vi "GuiRepository.vi"(0 "reference in":refnum<class "RemoteControl.lvclass">, 1 "Action(ReadRepository)":T1(ring), 5 "error in (no error)":errorcluster) -> (7 "QueueFromProcess":refnum<queue>, 9 "ProcessViRef":refnum<vi>, 11 "ProcessSyncQueue":refnum<queue>, 13 "EventFromProcess":refnum<user-event>, 14 "reference out":refnum<class "RemoteControl.lvclass">, 15 "EventsToProcess":refnum<user-event>, 17 "ProcessAlreadyStarted":bool, 19 "error out":errorcluster)   [LabVIEW 2012, in "RemoteControl.lvclass"]
uses:
  RemoteControl.lvclass
  Gui.ctl
  RemoteControl.lvclass/RemoteControl.ctl
  Gui.vi
panel:
  # "Use this indicator for sending messages to the Process VI"
  # "These indicators are used by the process VIs"
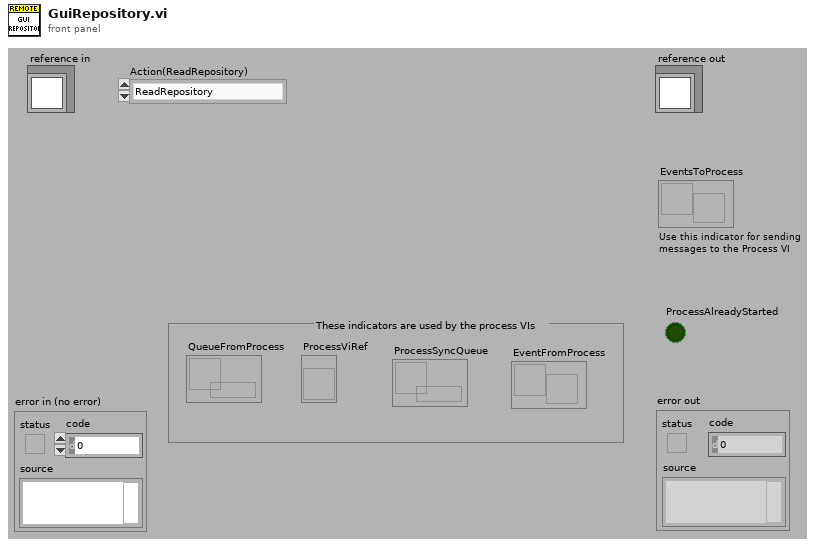
[diagram p1: front panel]
types:
  T1 = enum16{"ReadRepository", "CreateNew", "CreateOrLookUpExisting"}
  T2 = typedef "RemoteControl.lvclass/Gui.ctl" = cluster{"EventsToProcess":refnum<user-event>, "EventFromProcess":refnum<user-event>, "ProcessSyncQueue":refnum<queue>, "ProcessViRef":refnum<vi>, "QueueFromProcess":refnum<queue>}
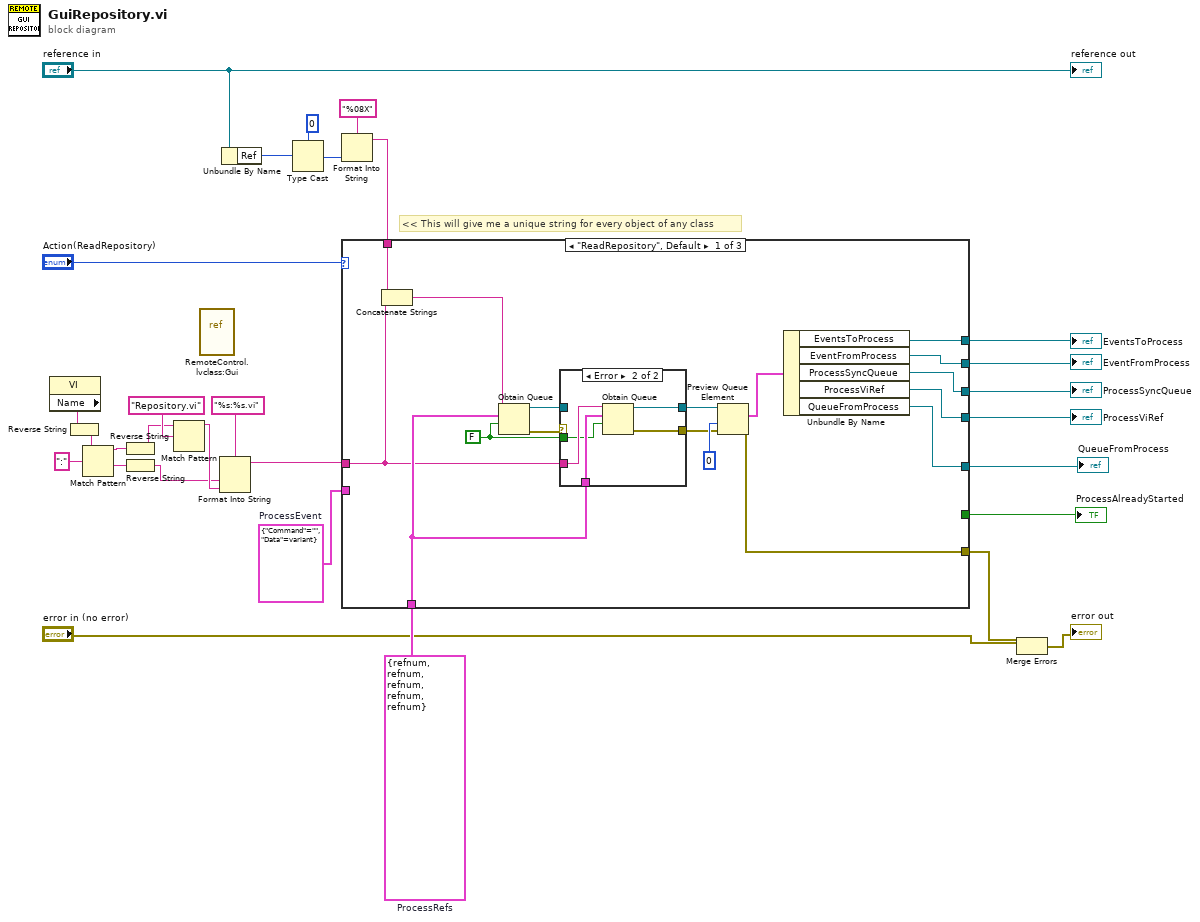
[diagram p0: block diagram]
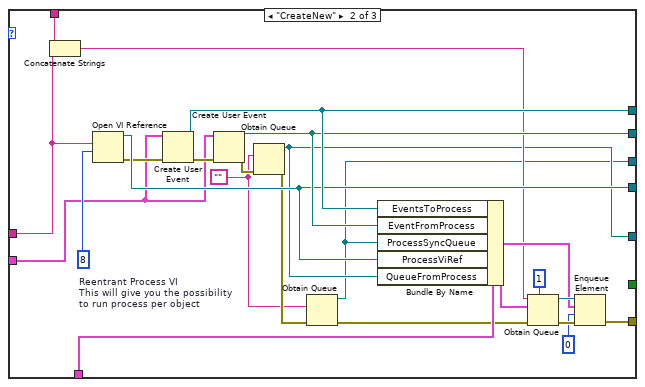
[diagram p3: hidden frame]
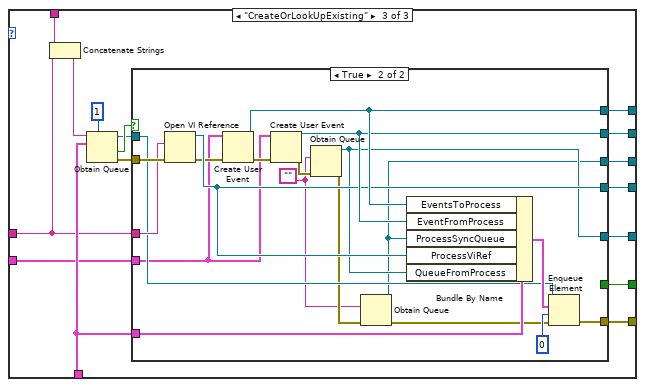
[diagram p4: hidden frame]
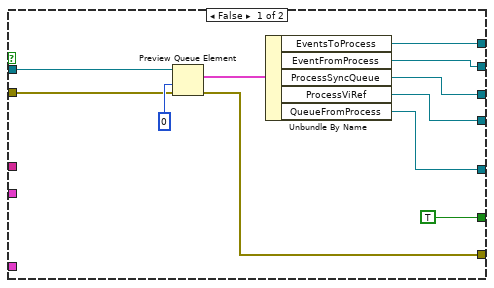
[diagram p5: hidden frame]
diagram:
  w13 = T2 {"EventsToProcess"=refnum, "EventFromProcess"=refnum, "ProcessSyncQueue"=refnum, "ProcessViRef"=refnum, "QueueFromProcess"=refnum}  # ProcessRefs
  w14 = cluster{"Command":string, "Data":variant} {"Command"="", "Data"=variant}  # ProcessEvent
  # "<< This will give me a unique string for every object of any class"
  n1 = property class="VI"() -> ("Name"=w20:string)  [unwired: 2 in, 2 out]
  n2 = Reverse String(1:w20) -> (0:w21:string)
  n3 = Match Pattern(string=w21, regular expression=":") -> (before substring=w25:string, after substring=w22:string)  [unwired: 1 in, 2 out]
  n4 = Reverse String(1:w25) -> (0:w26:string)
  n5 = Reverse String(1:w22) -> (0:w24:string)
  n6 = Match Pattern(string=w26, regular expression="Repository.vi") -> (before substring=w28:string)  [unwired: 1 in, 3 out]
  n7 = vi-ref "RemoteControl.lvclass:Gui.vi"() -> ()  [unwired: 1 out]
  n8 = Format Into String(format string="%s:%s.vi", w24, w28) -> (resulting string=w3:string)  [unwired: 2 in, 1 out]
  n9 = Unbundle By Name("reference in") -> ("Ref"=w15:u32)
  n10 = Type Cast(type=u32 0, x=w15) -> (*(type *) &x=w18:u32)
  n11 = Format Into String(format string="%08X", w18) -> (resulting string=w5:string)  [unwired: 2 in, 1 out]
  n12 = case shown="\"ReadRepository\", Default" "Action(ReadRepository)" {
    tunnel: [w42 w54 w90] -> w8
    tunnel: [w44 w76 w92] -> w6
    tunnel: [w43 w75 w91] -> w7
    tunnel: [w45 w74 w89] -> w9
    tunnel: w13 -> [w36 w64 w85]
    tunnel: w5 -> [w34 w63 w81]
    tunnel: [w41 w73 w88] -> w11
    tunnel: w3 -> [w33 w61 w80]
    tunnel: [_ _ w83] -> w10
    tunnel: w14 -> [_ w60 w78]
    tunnel: [w31 w58 w77] -> w1
    frame "ReadRepository", Default {
      w35 = FALSE ("create if not found? (T)")
      n13 = Concatenate Strings(w34, w33) -> (w32:string)
      n14 = Obtain Queue(name (unnamed)=w32, element data type=w36, create if not found? (T)=w35) -> (queue out=w38:refnum<queue>, error out=w40:errorcluster)  [unwired: 2 in, 1 out]
      n15 = case shown="Error" w40 {
        selector: w40 -> [w48 _]
        tunnel: [w48 w50] -> w39
        tunnel: w38 -> [w47 _]
        tunnel: [w47 w51] -> w37
        tunnel: w36 -> [_ w53]
        tunnel: w33 -> [_ w52]
        tunnel: w35 -> [_ w49]
        frame No Error {
        }
        frame Error {
          n16 = Obtain Queue(name (unnamed)=w52, element data type=w53, create if not found? (T)=w49) -> (queue out=w51:refnum<queue>, error out=w50:errorcluster)  [unwired: 2 in, 1 out]
        }
      }
      n17 = Preview Queue Element(queue=w37, timeout in ms (-1)=0, error in (no error)=w39) -> (element=w30:T2, error out=w41:errorcluster)  [unwired: 2 out]
      n18 = Unbundle By Name(w30) -> ("EventsToProcess"=w44:refnum<user-event>, "EventFromProcess"=w43:refnum<user-event>, "ProcessSyncQueue"=w42:refnum<queue>, "ProcessViRef"=w45:refnum<vi>, "QueueFromProcess"=w31:refnum<queue>)
    }
    frame "CreateNew" {
      w55 = ""
      w70 = 8  # Reentrant Process VI This will give you the possibility to run process per object
      n19 = Concatenate Strings(w63, w61) -> (w62:string)
      n20 = Open VI Reference(vi path=w61, options=w70) -> (vi reference=w74:refnum<vi>, error out=w71:errorcluster)  [unwired: 4 in]
      n21 = Create User Event(user event datatype=w60, error in=w71) -> (user event=w76:refnum<user-event>, error out=w72:errorcluster)
      n22 = Create User Event(user event datatype=w60, error in=w72) -> (user event=w75:refnum<user-event>, error out=w59:errorcluster)
      n23 = Obtain Queue(element data type=w55, error in (no error)=w59) -> (queue out=w58:refnum<queue>, error out=w57:errorcluster)  [unwired: 3 in, 1 out]
      n24 = Obtain Queue(element data type=w55, error in (no error)=w57) -> (queue out=w54:refnum<queue>, error out=w56:errorcluster)  [unwired: 3 in, 1 out]
      n25 = Bundle By Name(cluster=w64, "EventsToProcess"=w76, "EventFromProcess"=w75, "ProcessSyncQueue"=w54, "ProcessViRef"=w74, "QueueFromProcess"=w58) -> (w67:T2)
      n26 = Obtain Queue(max queue size (-1, unlimited)=1, name (unnamed)=w62, element data type=w67, error in (no error)=w56) -> (queue out=w69:refnum<queue>, error out=w68:errorcluster)  [unwired: 1 in, 1 out]
      n27 = Enqueue Element(queue=w69, element=w67, timeout in ms (-1)=0, error in (no error)=w68) -> (error out=w73:errorcluster)  [unwired: 2 out]
    }
    frame "CreateOrLookUpExisting" {
      n28 = Concatenate Strings(w81, w80) -> (w79:string)
      n29 = Obtain Queue(max queue size (-1, unlimited)=1, name (unnamed)=w79, element data type=w85) -> (queue out=w86:refnum<queue>, created new?=w87:bool, error out=w84:errorcluster)  [unwired: 2 in]
      n30 = case shown="True" w87 {
        tunnel: [w103 w122] -> w92
        tunnel: [w102 w121] -> w91
        tunnel: [w101 w104] -> w90
        tunnel: [w100 w120] -> w89
        tunnel: [w96 w119] -> w88
        tunnel: w85 -> [_ w118]
        tunnel: w84 -> [w97 w113]
        tunnel: w80 -> [_ w112]
        tunnel: w86 -> [w98 w111]
        tunnel: [TRUE _] -> w83
        tunnel: w78 -> [_ w110]
        tunnel: [w93 w108] -> w77
        frame False {
          n31 = Preview Queue Element(queue=w98, timeout in ms (-1)=0, error in (no error)=w97) -> (element=w95:T2, error out=w96:errorcluster)  [unwired: 2 out]
          n32 = Unbundle By Name(w95) -> ("EventsToProcess"=w103:refnum<user-event>, "EventFromProcess"=w102:refnum<user-event>, "ProcessSyncQueue"=w101:refnum<queue>, "ProcessViRef"=w100:refnum<vi>, "QueueFromProcess"=w93:refnum<queue>)
        }
        frame True {
          w105 = ""
          n33 = Open VI Reference(vi path=w112, error in (no error)=w113) -> (vi reference=w120:refnum<vi>, error out=w116:errorcluster)  [unwired: 4 in]
          n34 = Create User Event(user event datatype=w110, error in=w116) -> (user event=w122:refnum<user-event>, error out=w117:errorcluster)
          n35 = Create User Event(user event datatype=w110, error in=w117) -> (user event=w121:refnum<user-event>, error out=w109:errorcluster)
          n36 = Obtain Queue(element data type=w105, error in (no error)=w109) -> (queue out=w108:refnum<queue>, error out=w107:errorcluster)  [unwired: 3 in, 1 out]
          n37 = Obtain Queue(element data type=w105, error in (no error)=w107) -> (queue out=w104:refnum<queue>, error out=w106:errorcluster)  [unwired: 3 in, 1 out]
          n38 = Bundle By Name(cluster=w118, "EventsToProcess"=w122, "EventFromProcess"=w121, "ProcessSyncQueue"=w104, "ProcessViRef"=w120, "QueueFromProcess"=w108) -> (w115:T2)
          n39 = Enqueue Element(queue=w111, element=w115, timeout in ms (-1)=0, error in (no error)=w106) -> (error out=w119:errorcluster)  [unwired: 2 out]
        }
      }
    }
  }
  "ProcessSyncQueue" <- w8
  "EventsToProcess" <- w6
  "EventFromProcess" <- w7
  "ProcessViRef" <- w9
  "ProcessAlreadyStarted" <- w10
  "QueueFromProcess" <- w1
  n40 = Merge Errors("error in (no error)", w11) -> (→"error out":errorcluster)
  "reference out" <- "reference in"
